vi "INIdialog.vi"(8 "Error In":errorcluster) -> (0 "Error Out":errorcluster, 3 "ServerINI":T1={"ClientTimeout (s)"=30, "LogPath"=path "C:/Users/jgoebel/Documents/GitHub/AEDashboard/ServerLib/Data/ServerLog.tdms", "ErrorsToIgnore"=[], "OracleData"={"DBname"="", "User"="", "Password"=""}})   [LabVIEW 2017, in "Server.lvlib"]
doc: "Popup Dialog!\nThis VI accepts User Input for the INI Data in case the INI file wasnt read properly. It then passes this Data and creates a new INI-File with this Data. If the User chooses to cancel this dialog it will output an error and stop the application."
uses:
  Server.lvlib
  TypeDefs/ServerINI.ctl
  SubLibs/Oracle/OracleData.ctl
  <vilib>/Utility/error.llb/Error Cluster From Error Code.vi
  <vilib>/ErrorRing/Error Ring.xnode
  SubLibs/Oracle/Oracle.lvlib
panel:
  in  "Cancel Button":bool
  in  "OK Button":bool
  in  "ServerINI 2":T1={"ClientTimeout (s)"=30, "LogPath"=path "C:/Users/jgoebel/Documents/GitHub/AEDashboard/ServerLib/Data/ServerLog.tdms", "ErrorsToIgnore"=[], "OracleData"={"DBname"="", "User"="", "Password"=""}}
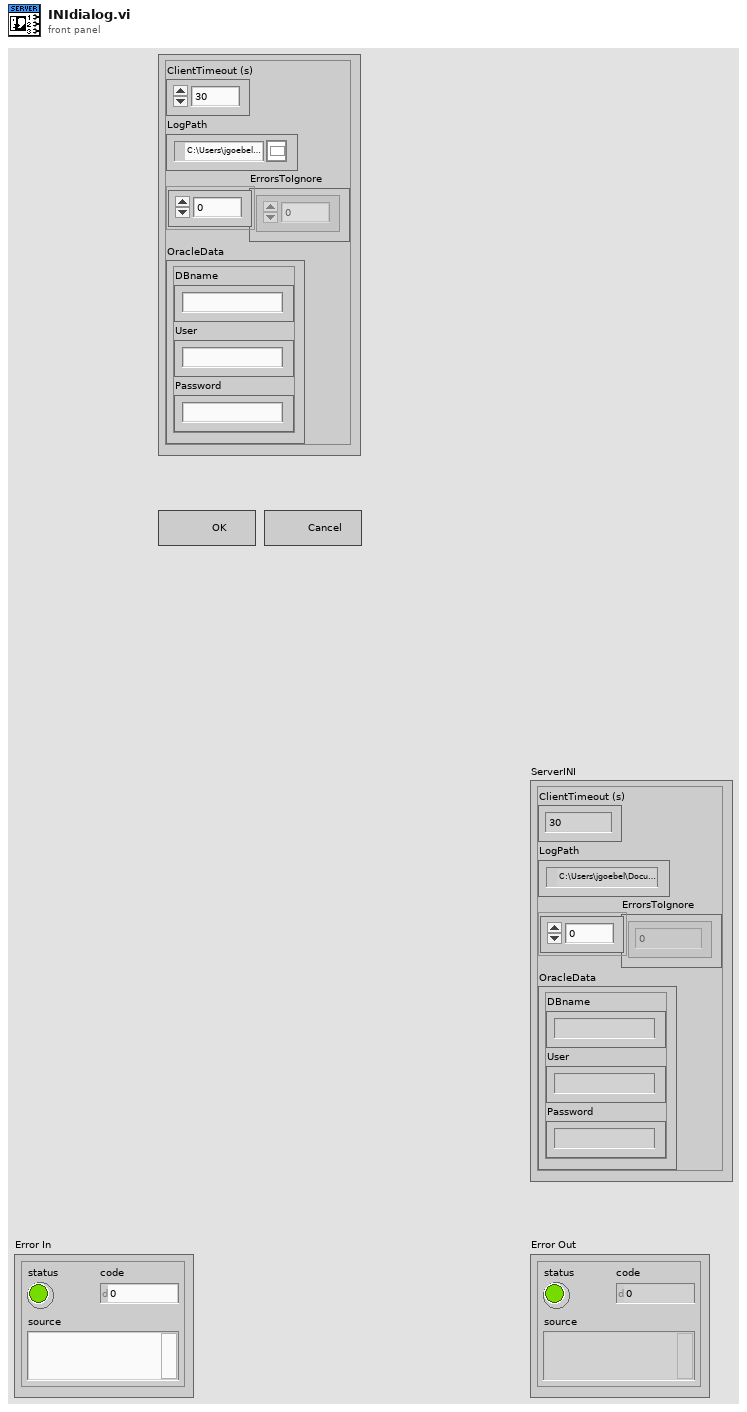
[diagram p1: front panel]
types:
  T1 = typedef "Server.lvlib/ServerINI.ctl" = cluster{"ClientTimeout (s)":u32, "LogPath":path, "ErrorsToIgnore":i32[], "OracleData":T2}
  T2 = typedef "Server.lvlib/Oracle.lvlib/OracleData.ctl" = cluster{"DBname":string, "User":string, "Password":string}
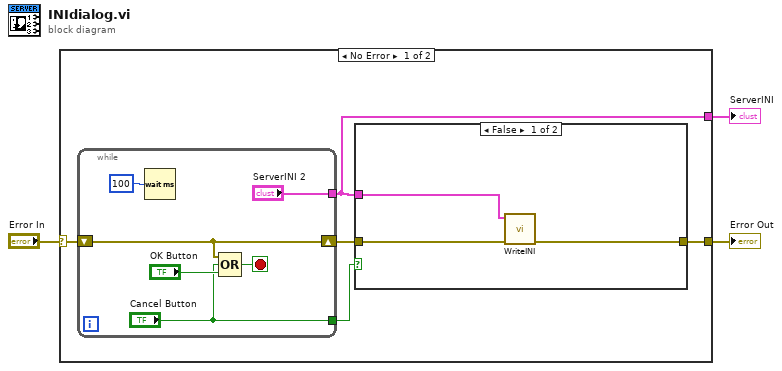
[diagram p0: block diagram]
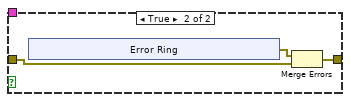
[diagram p2: hidden frame]
diagram:
  n1 = case shown="No Error" "Error In" {
    selector: "Error In" -> [w8 w26]
    tunnel: [w6 w26] -> w2
    tunnel: [w4 _] -> w1
    frame No Error {
      n2 = while {
        shift-right: [w24] -> w7
        shift-left: w8 -> [w24]
        tunnel: ["Cancel Button"] -> w5
        tunnel: ["ServerINI 2"] -> w4
        stop <- w23 stop-if-true
        n3 = Wait (ms)(milliseconds to wait=u32 100) -> ()  [unwired: 1 out]
        n4 = Compound Arithmetic op=OR(w24, "Cancel Button", "OK Button") -> (w23:bool)
      }
      n5 = case shown="False" w5 {
        tunnel: w7 -> [w11 w14]
        tunnel: [w10 w13] -> w6
        tunnel: w4 -> [w9 _]
        frame False {
          n6 = call "WriteINI.vi"("Error In"=w11, "ServerINI"=w9) -> ("Error Out"=w10:errorcluster)  [unwired: 9 in]
        }
        frame True {
          n7 = xnode "Error Ring"() -> ("error out"=w12:errorcluster)
          n8 = Merge Errors(w12, w14) -> (w13:errorcluster)
        }
      }
    }
    frame Error {
    }
  }
  "Error Out" <- w2
  "ServerINI" <- w1
